vi "label ROI.vi"(8 "error in (no error)":errorcluster caption="错误输入（无错误）", 9 "beads track":T1[](array[typedef]) {"centroid"."Y Centroid" format="%.2f"; "centroid"."X Centroid" format="%.2f"; "ROI Des out"."Contours"."Type" items=["No Selection", "Point", "Line", "Rectangle", "Oval", "Polygon", "Freehand Region", "Annulus", "Unused2", "Unused3", "Broken Line", "Freehand Line", "Rotated Rectangle"]}, 10 "beads info":T3[](array[typedef]), 11 "CCD image ref":T4) -> (0 "error out":errorcluster caption="错误输出", 3 "labeled Image Out":T4)   [LabVIEW 2017]
doc: "本Vi的功能是输入每个ROI的图心位置，在每个ROI的图心位置上标明相应的编号。\n输入：CCD image ref , 注意，是采集的CCD图像的引用，不是任何一个ROI的图像引用，输错会造成坐标出错。\ncentroid array： 各个ROI 的图心位置组成的矩阵，一般是从tracking 循环中直接输出的索引。\n输出：labeled image ref ，注意，如果有多个地方要编号，这里的image 已经通过移位寄存器进行了多次标记，所以输出的图像是有好几个标记的，不会像之前每张图只有一个地方编号，编号多了会导致闪烁。这里是每个ROI都同时编号的。\n可以在程序框图里修改颜色，字号等等。"
uses:
  <vilib>/vision/Image Controls.llb/IMAQ Image.ctl
  control/bead info.ctl
  control/Bead track.ctl
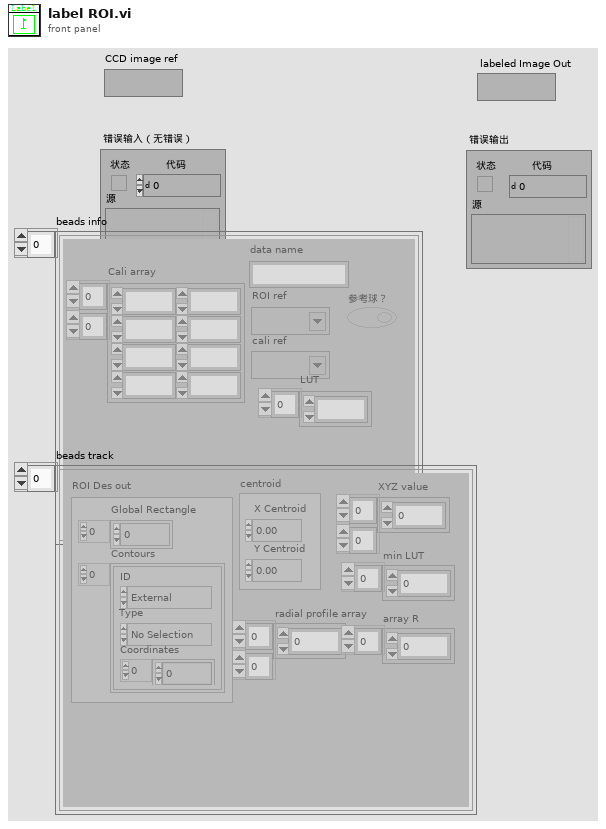
[diagram p1: front panel]
types:
  T1 = typedef "Bead track.ctl" = cluster{"XYZ value":dbl[][], "radial profile array":dbl[][], "min LUT":dbl[], "ROI Des out":T2, "array R":dbl[], "centroid":cluster{"X Centroid":sgl, "Y Centroid":sgl}}
  T2 = typedef "ROI Descriptor" = cluster{"Global Rectangle":i32[], "Contours":cluster{"ID":enum32{"External", "Internal"}, "Type":u32, "Coordinates":i32[]}[]}
  T3 = typedef "bead info.ctl" = cluster{"data name":string, "ROI ref":T4, "cali ref":T4, "参考球？":bool, "LUT":dbl[], "Cali array":dbl[][], "修正次数":i32, "R_step":dbl, "sample(quar)":i32}
  T4 = typedef "IMAQ Image.ctl" = refnum<image>
  T5 = cluster{"Desired Font (Application)":enum16{"User-specified Font", "Application Font", "System Font", "Dialog Font"}, "[User-specified Font]":cluster{"Font Name":string, "Size":i16, "Strikeout?":bool, "Italic?":bool, "Underline?":bool, "Outline?":bool, "Shadow?":bool, "Bold?":bool, "Rotation Angle":dbl}, "Horizontal Alignment":i16, "Vertical Alignment":i16}
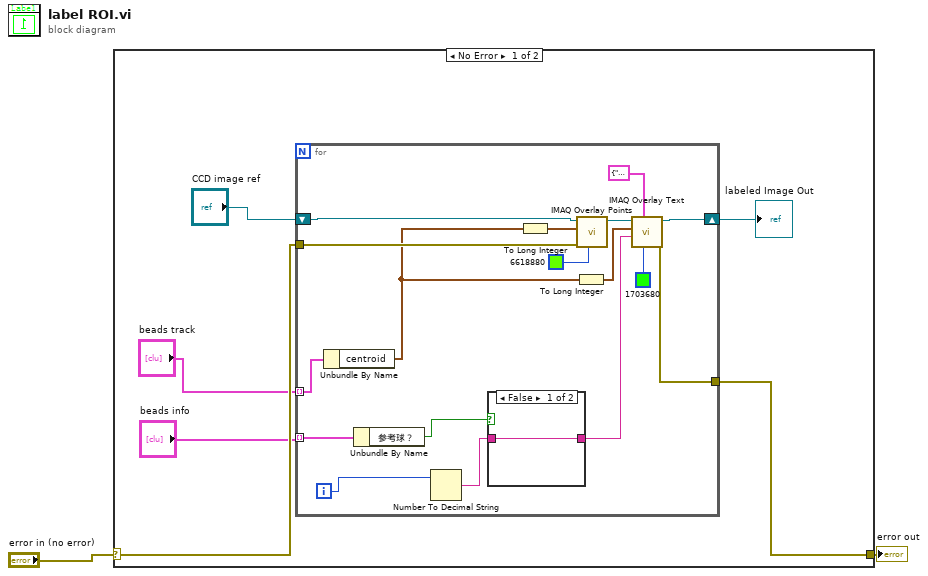
[diagram p0: block diagram]
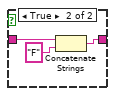
[diagram p2: hidden frame]
diagram:
  n1 = case shown="No Error" "error in (no error)" {
    selector: "error in (no error)" -> [w7 w30]
    tunnel: [w8 w30] -> w1
    frame No Error {
      n2 = for {
        tunnel: [w24] -> w8
        tunnel: w7 -> [w19]
        shift-right: [w23] -> w6
        shift-left: "CCD image ref" -> [w22]
        tunnel: "beads track" -> [w15] mode=indexing
        tunnel: "beads info" -> [w11] mode=indexing
        i -> [w12]
        n3 = Unbundle By Name(w15) -> ("centroid"=w9:cluster{"X Centroid":sgl, "Y Centroid":sgl})
        n4 = Unbundle By Name(w11) -> ("参考球？"=w10:bool)
        n5 = Number To Decimal String(number=w12) -> (decimal integer string=w17:string)  [unwired: 1 in]
        n6 = case shown="False" w10 {
          tunnel: w17 -> [w26 w29]
          tunnel: [w26 w27] -> w16
          frame False {
          }
          frame True {
            n7 = Concatenate Strings(w29, "F" ("字符串")) -> (w27:string)
          }
        }
        n8 = To Long Integer(number=w9) -> (32bit integer=w13:cluster{"X Centroid":i32, "Y Centroid":i32})
        n9 = To Long Integer(number=w9) -> (32bit integer=w14:cluster{"X Centroid":i32, "Y Centroid":i32})
        n10 = call "IMAQ Overlay Points"("Color"=u32 6618880, "error in (no error)"=w19, "Point"=w13, "Image"=w22) -> ("Image Out"=w20:T4)  [unwired: 6 in, 1 out]
        n11 = call "IMAQ Overlay Text"("Text Color (black)"=u32 1703680, "Font, Size & Style"=T5 {"Desired Font (Application)"=enum."Application Font", "[User-specified Font]"={"Font Name"="", "Size"=36, "Strikeout?"=FALSE, "Italic?"=FALSE, "Underline?"=FALSE, "Outline?"=FALSE, "Shadow?"=FALSE, "Bold?"=FALSE, "Rotation Angle"=0.0}, "Horizontal Alignment"=0, "Vertical Alignment"=0}, "String"=w16, "Origin"=w14, "Image"=w20) -> ("error out"=w24:errorcluster, "Image Out"=w23:T4)  [unwired: 5 in]
      }
      "labeled Image Out" <- w6
    }
    frame Error {
    }
  }
  "error out" <- w1
